vi "HardPass.vi"(0 "Password":string, 11 "error in (no error)":errorcluster) -> (4 "Password out":string, 8 "Hard enough?":bool, 14 "What is missed":string, 15 "error out":errorcluster)   [LabVIEW 2012]
panel:
  out "Mayus":bool
  out "Letra":bool
  out "num":bool
  out "simbol":bool
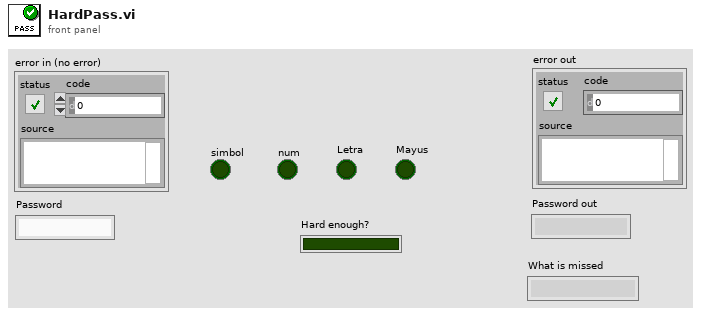
[diagram p1: front panel]
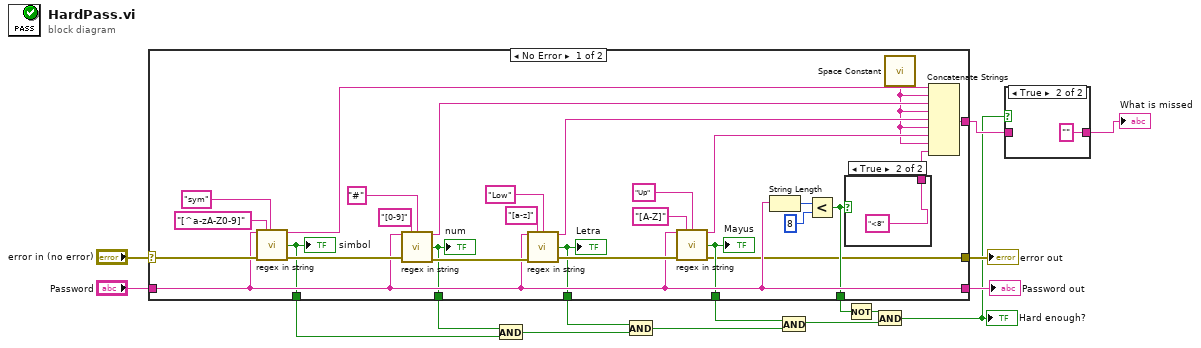
[diagram p0: block diagram]
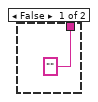
[diagram p3: hidden frame]
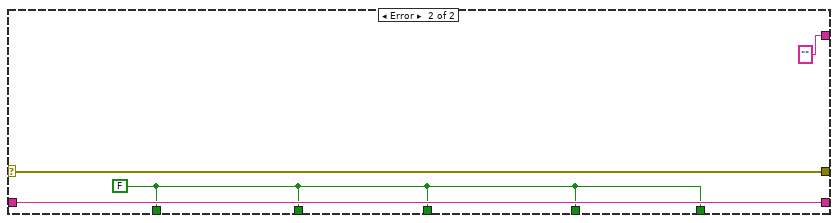
[diagram p4: hidden frame]
diagram:
  n1 = case shown="No Error" "error in (no error)" {
    selector: "error in (no error)" -> [w44 w50]
    tunnel: "Password" -> [w36 w49]
    tunnel: [w24 w50] -> w14
    tunnel: [w36 w49] -> w13
    tunnel: [w33 w48] -> w4
    tunnel: [w32 w48] -> w10
    tunnel: [w31 w48] -> w8
    tunnel: [w30 w48] -> w7
    tunnel: [w29 w48] -> w6
    tunnel: [w22 ""] -> w2
    frame No Error {
      n2 = call "regex in string.vi"("string"=w36, "regular expression"="[^a-zA-Z0-9]", "Error String"="sym" ("source"), "error in (no error)"=w44) -> ("Error String Out"=w21:string, "reg ex is in the string?"=w29:bool, "error out"=w37:errorcluster)  [unwired: 9 in]
      "simbol" <- w29
      n3 = call "regex in string.vi"("string"=w36, "regular expression"="[0-9]", "Error String"="#" ("source"), "error in (no error)"=w37) -> ("Error String Out"=w20:string, "reg ex is in the string?"=w30:bool, "error out"=w38:errorcluster)  [unwired: 9 in]
      "num" <- w30
      n4 = call "regex in string.vi"("string"=w36, "regular expression"="[a-z]", "Error String"="Low" ("source"), "error in (no error)"=w38) -> ("Error String Out"=w23:string, "reg ex is in the string?"=w31:bool, "error out"=w39:errorcluster)  [unwired: 9 in]
      "Letra" <- w31
      n5 = call "regex in string.vi"("string"=w36, "regular expression"="[A-Z]", "Error String"="Up" ("source"), "error in (no error)"=w39) -> ("Error String Out"=w18:string, "reg ex is in the string?"=w32:bool, "error out"=w24:errorcluster)  [unwired: 9 in]
      "Mayus" <- w32
      n6 = String Length(string=w36) -> (length=w35:i32)
      n7 = Less?(x=w35, y=8) -> (x < y?=w33:bool)
      n8 = case shown="True" w33 {
        tunnel: ["" "<8" ("source")] -> w19
        frame False {
        }
        frame True {
        }
      }
      n9 = call <vilib>:"Space Constant.vi"() -> ("String"=w17:string)
      n10 = Concatenate Strings(w21, w17, w20, w17, w23, w17, w18, w17, w19) -> (w22:string)
    }
    frame Error {
      w48 = FALSE
    }
  }
  "error out" <- w14
  "Password out" <- w13
  n11 = And(x=w7, y=w6) -> (x .and. y?=w9:bool)
  n12 = And(x=w8, y=w9) -> (x .and. y?=w11:bool)
  n13 = And(x=w10, y=w11) -> (x .and. y?=w12:bool)
  n14 = Not(x=w4) -> (.not. x?=w5:bool)
  n15 = And(x=w5, y=w12) -> (x .and. y?=w1:bool)
  "Hard enough?" <- w1
  n16 = case shown="True" w1 {
    tunnel: [w51 ""] -> w3
    tunnel: w2 -> [w51 _]
    frame False {
    }
    frame True {
    }
  }
  "What is missed" <- w3
